vi "String to Ring Converter.vi"(10 "Control Name":string, 11 "Ring Control":refnum<vi>) -> (3 "Value":i32)   [LabVIEW 2021, in "User Interface.lvlib"]
uses:
  User Interface.lvlib
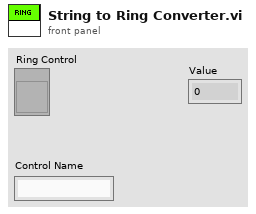
[diagram p1: front panel]
types:
  T1 = typedef "LVStringsAndValuesArrayTypeDef_I32.ctl" = cluster{"String":string, "Value":i32}[]
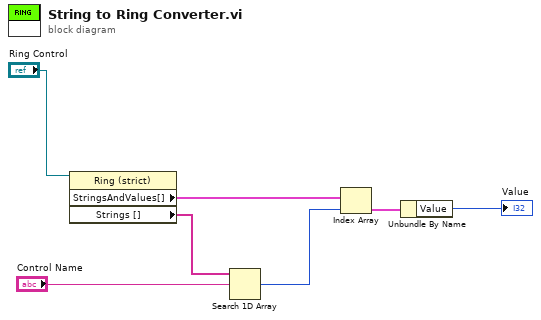
[diagram p0: block diagram]
diagram:
  n1 = property class="Ring (strict)"(reference="Ring Control") -> ("StringsAndValues[]"=w6:T1, "Strings []"=w5:string[])  [unwired: 1 in, 2 out]
  n2 = Search 1D Array(1D array=w5, element="Control Name") -> (index of element=w3:i32)  [unwired: 1 in]
  n3 = Index Array(array=w6, index=w3) -> (element=w2:cluster{"String":string, "Value":i32})
  n4 = Unbundle By Name(w2) -> ("Value"=→"Value":i32)
